vi "Pilot-Screen.vi"() -> ()   [LabVIEW 2018]
uses:
  <vilib>/userdefined/High Color/IMAQdx.ctl
  <vilib>/vision/Shape Detection.llb/ShapeDetectionMatchOptions.ctl
  <vilib>/vision/Pattern Matching.llb/IMAQ Match Range Setting.ctl
  <vilib>/express/express arith-compare/Formula/XNode/ExpressFormulaBlockNode.xnode
  <vilib>/vision/driver/NI_Vision_Acquisition_Software.lvlib
  <vilib>/MakerHub/LINX/LMH-LINX.lvlib
  <vilib>/vision/NI_Vision_Development_Module.lvlib
panel:
  in  "Tab Control":enum32{"Cannon calculations", "Shape Detection"}(tab)
  out "lift capability of ROV":dbl format="%#.1f"
  out "String 8":string
  in  "Cannon Volume":dbl format="%#.1f"
  out "Scaled Distance":dbl format="%#.1f"
  in  "Real Distance":dbl format="%#_6f"
  in  "Set Refrence":bool
  in  "Stop 2":bool
  out "Cannon Weight":dbl format="%#.1f"
  out "String 6":string
  out "String 7":string
  in  "Composition":u16(ring) items=["Select"=0, "AF"=8030, "Else"=7870]
  out "ROV Can Lift?":bool
  out "Snapshot":T1(plugin-control)
  out "String":string
  out "String 2":string
  out "String 4":string
  out "String 5":string
  in  "R1 2":dbl format="%#.1f"
  in  "R2 2":dbl format="%#.1f"
  in  "R3 2":dbl format="%#.1f"
  in  "L 2":bool
  in  "R1":bool
  in  "R2":bool
  in  "R3":bool
  in  "L":dbl format="%#.1f"
  out "Snapshot 2":T1(plugin-control)
  out "Done":bool
  out "Lines":i32
  out "Triangles":i32
  out "Squares":i32
  out "Circles":i32
  out "Objects":i32
  in  "Start Detecting":bool
  out "measurment Video":T1(plugin-control)
  in  "Scaled Pixels":dbl
  in  "Real Pixels":dbl
  in  "measurment camera":T2
  in  "Stop":bool
  in  "Gribber":T2="cam7"
  out "Loop Rate (Hz)":u32
  out "Grebber Camera":T1(plugin-control)
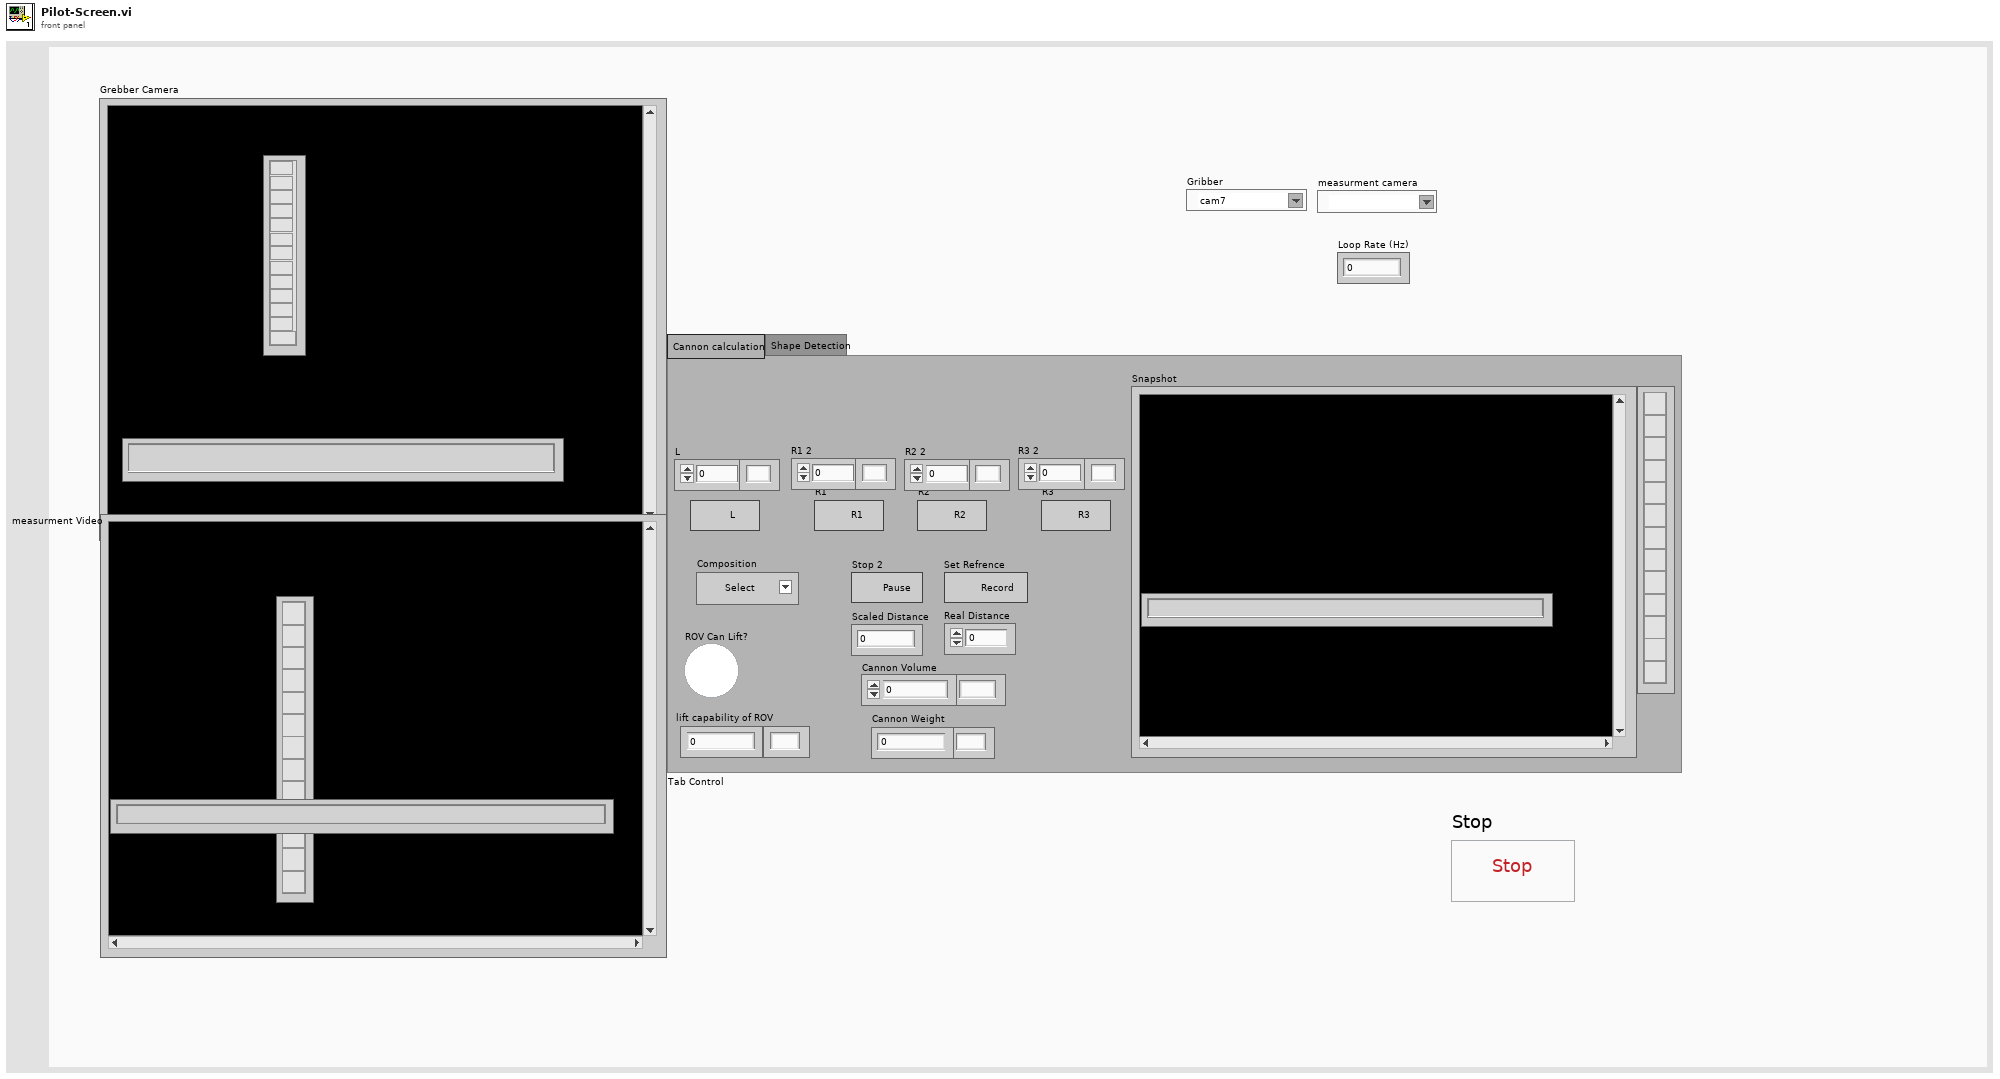
[diagram p1: front panel]
types:
  T1 = typedef "IMAQ Image.ctl" = refnum<image>
  T2 = typedef "IMAQdx.ctl" = refnum<k21>
  T3 = typedef "Image Type" = u32
  T4 = typedef "ShapeDetectionMatchOptions.ctl" = cluster{"Rotation":bool, "Scale":bool, "Occlusion":bool, "Range Settings":T5[]}
  T5 = typedef "IMAQ Match Range Setting.ctl" = cluster{"Match Constraints":u32, "Min":dbl, "Max":dbl}
  T6 = cluster{"Objects":u16, "Threshold":i32, "Reject Border":bool, "Fill Holes":bool, "Min Object Size":bool, "Min Size":i32, "Max Object Size":bool, "Max Size":i32, "Show Search Area":bool, "Show Center":bool, "Show Bounding Box":bool}
  T7 = cluster{"Global Rectangle":i32[], "Contours":cluster{"Contour Type":u32, "ROI Type":u32, "Points":i32[]}[]}
  T8 = typedef "IMAQ Line" = cluster{"Start X":i32, "Start Y":i32, "End X":i32, "End Y":i32}
  T9 = typedef "IMAQ Rectangle" = cluster{"Left":i32, "Top":i32, "Right":i32, "Bottom":i32, "Rotation":dbl}
  T10 = cluster{"Object Center":cluster{"X":sgl, "Y":sgl}, "Bounding Box":cluster{"X Left":i32, "Y Top":i32, "X Right":i32, "Y Bottom":i32}, "Area":sgl, "Orientation":sgl, "Aspect Ratio":sgl, "Nb Holes":i32}[]
  T11 = cluster{"Object Center":cluster{"X":sgl, "Y":sgl}, "Bounding Box":cluster{"X Left":i32, "Y Top":i32, "X Right":i32, "Y Bottom":i32}, "Area":sgl, "Orientation":sgl, "Aspect Ratio":sgl, "Nb Holes":i32}
  T12 = typedef "ROI Descriptor" = cluster{"Global Rectangle":i32[], "Contours":cluster{"ID":enum32{"External", "Internal"}, "Type":u32, "Coordinates":i32[]}[]}
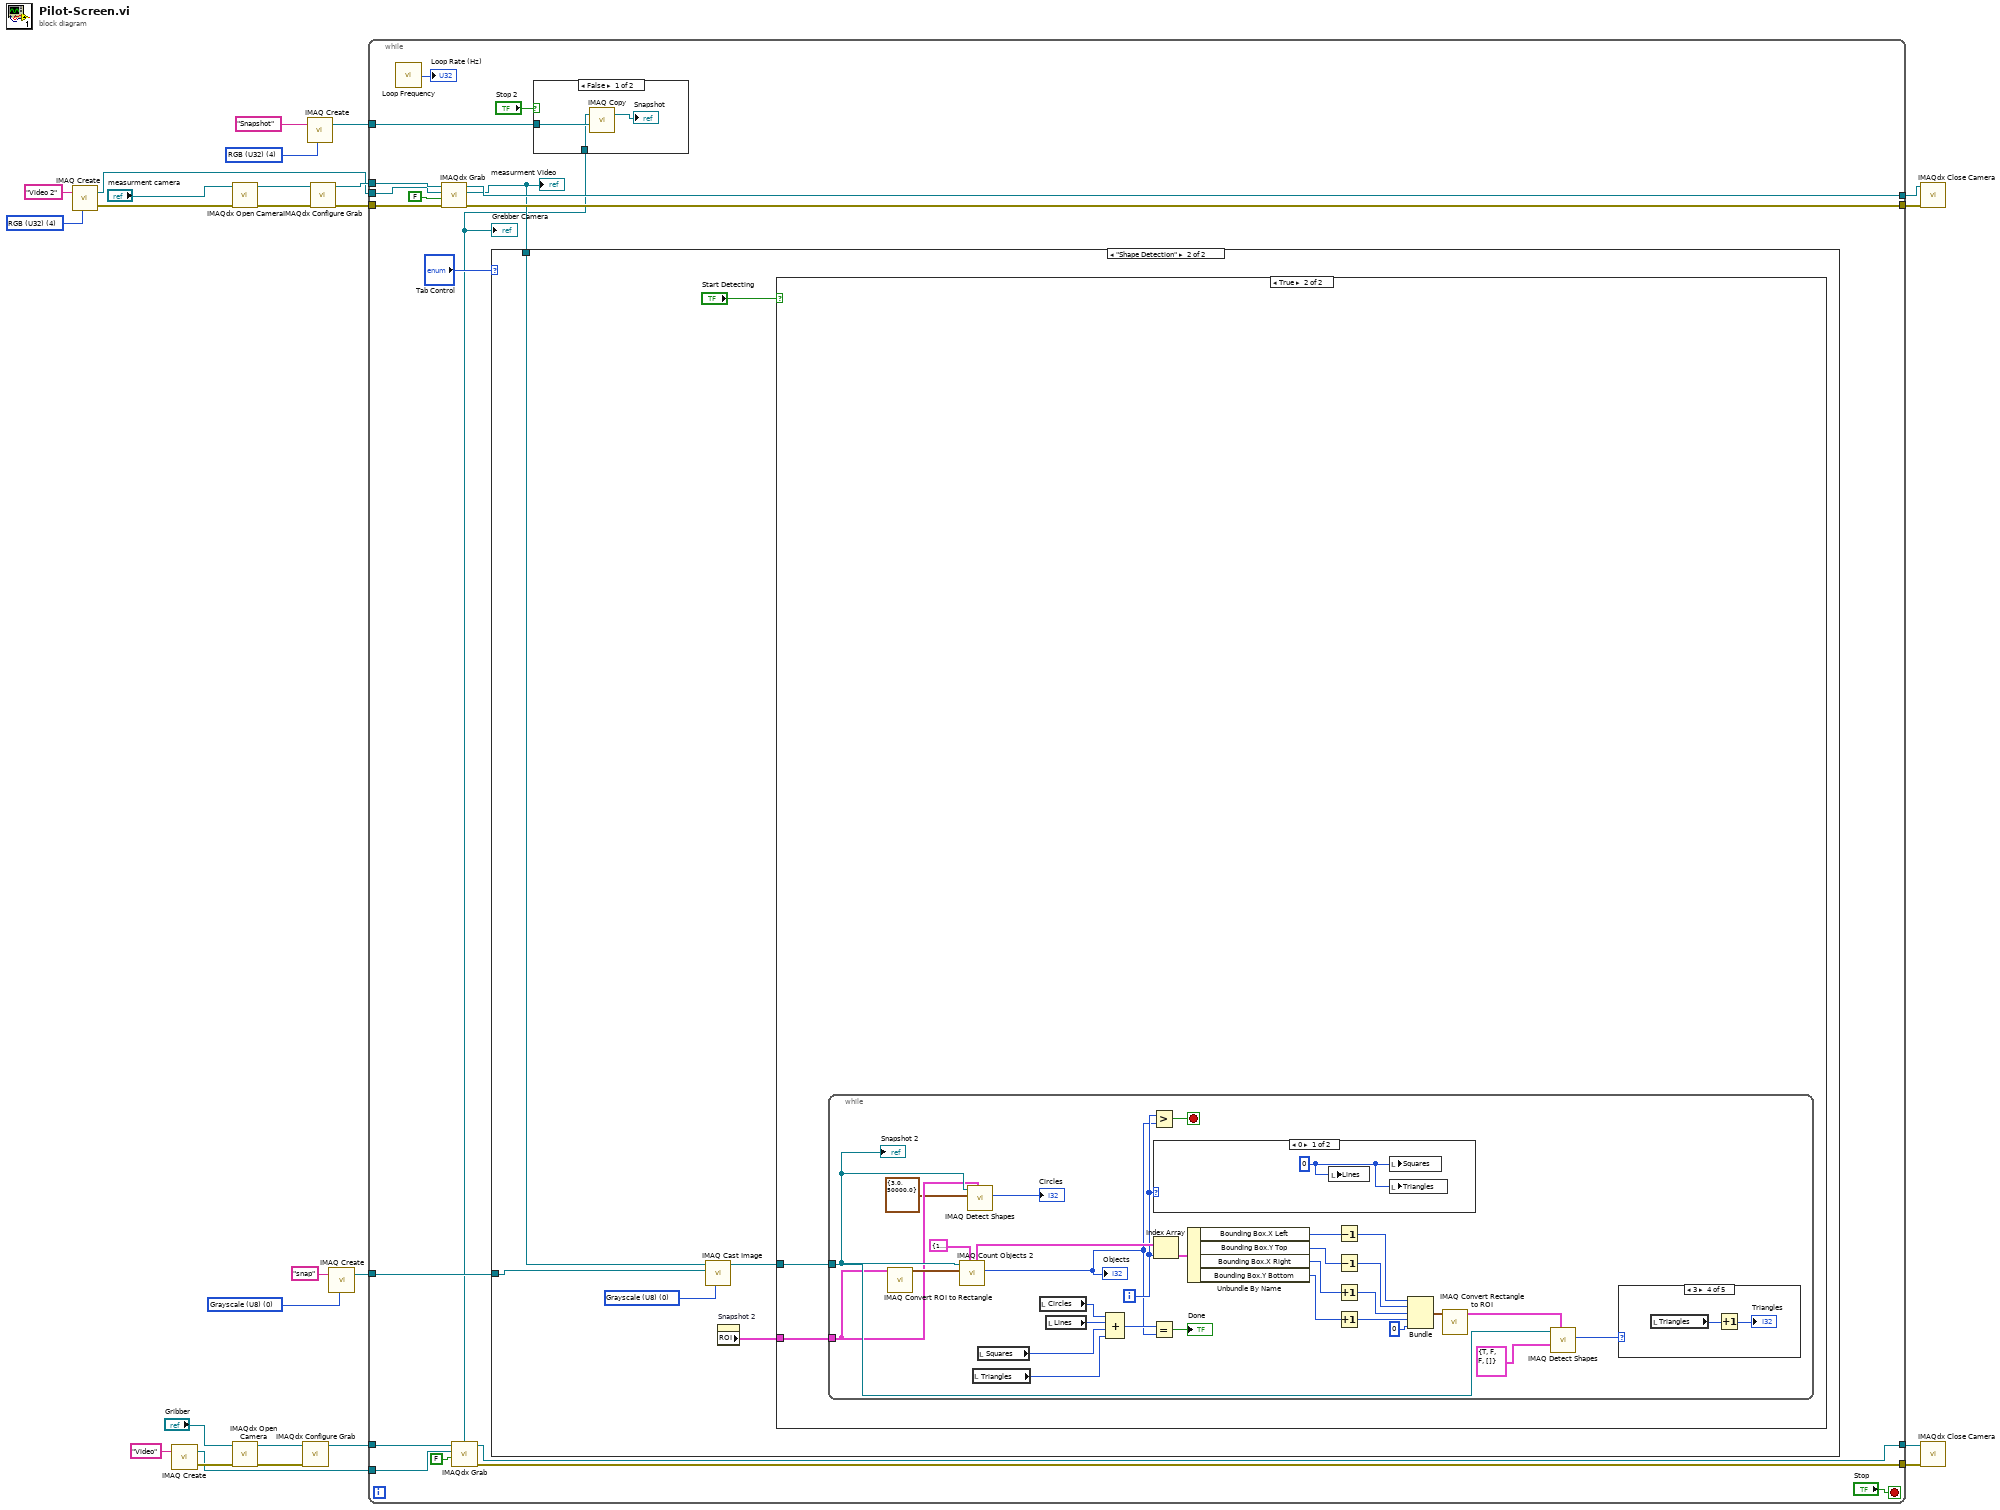
[diagram p0: block diagram]
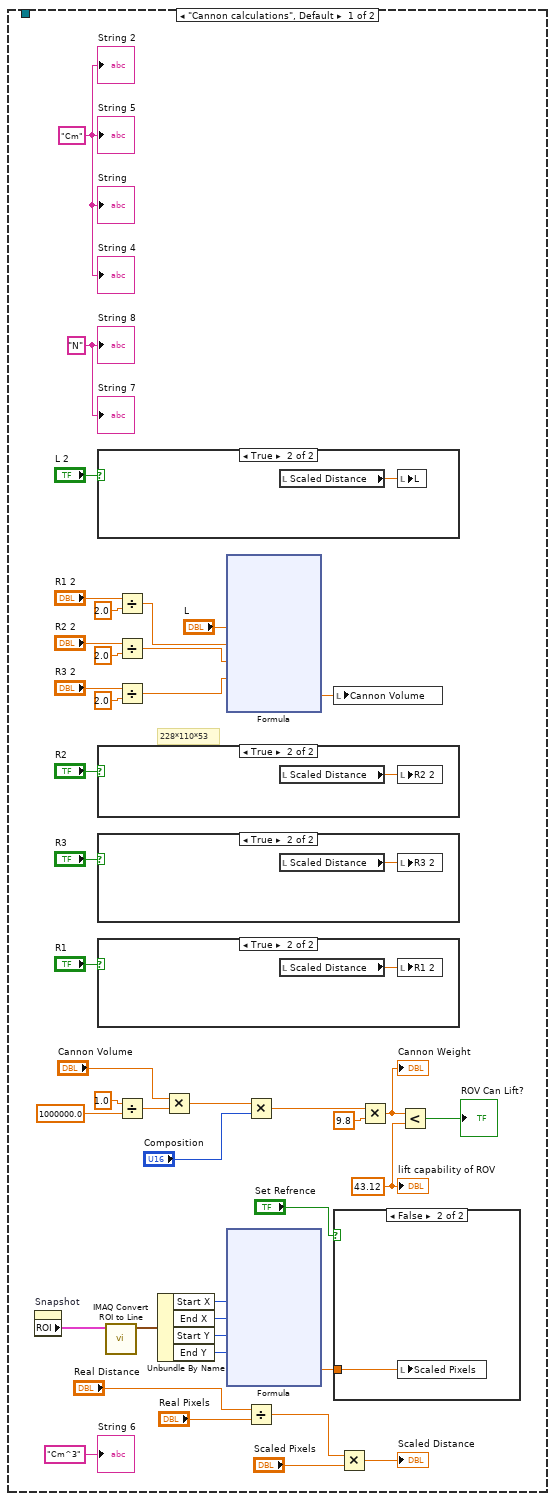
[diagram p2: hidden frame]
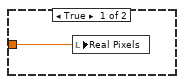
[diagram p7: hidden frame]
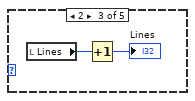
[diagram p11: hidden frame]
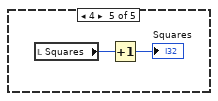
[diagram p12: hidden frame]
diagram:
  w3 = T3 0 items=["Grayscale (U8)", "Grayscale (I16)", "Grayscale (SGL)", "Complex (CSG)", "RGB (U32)", "HSL (U32)", "RGB (U64)", "Grayscale (U16)"] ("Image Type")
  w15 = T3 4 items=["Grayscale (U8)", "Grayscale (I16)", "Grayscale (SGL)", "Complex (CSG)", "RGB (U32)", "HSL (U32)", "RGB (U64)", "Grayscale (U16)"] ("Image Type")
  w13 = T3 4 items=["Grayscale (U8)", "Grayscale (I16)", "Grayscale (SGL)", "Complex (CSG)", "RGB (U32)", "HSL (U32)", "RGB (U64)", "Grayscale (U16)"] ("Image Type")
  n1 = call "IMAQ Create"("Image Name"="Video 2", "Image Type"=w13) -> ("New Image"=w8:T1, "error out"=w17:errorcluster)  [unwired: 2 in, 1 out]
  n2 = call "IMAQ Create"("Image Name"="Video") -> ("New Image"=w22:T1, "error out"=w26:errorcluster)  [unwired: 3 in, 1 out]
  n3 = call <vilib>:"IMAQdx Open Camera.vi"("error in"=w17, "Session In"="measurment camera") -> ("error out"=w12:errorcluster, "Session Out"=w11:T2)  [unwired: 8 in]
  n4 = call <vilib>:"IMAQdx Open Camera.vi"("error in"=w26, "Session In"="Gribber") -> ("error out"=w25:errorcluster, "Session Out"=w24:T2)  [unwired: 8 in]
  n5 = call <vilib>:"IMAQdx Configure Grab.vi"("error in"=w25, "Session In"=w24) -> ("Session Out"=w21:T2)  [unwired: 8 in, 1 out]
  n6 = call "IMAQ Create"("Image Name"="Snapshot", "Image Type"=w15) -> ("New Image"=w7:T1)  [unwired: 3 in, 1 out]
  n7 = call <vilib>:"IMAQdx Configure Grab.vi"("error in"=w12, "Session In"=w11) -> ("error out"=w9:errorcluster, "Session Out"=w10:T2)  [unwired: 8 in]
  n8 = call "IMAQ Create"("Image Name"="snap", "Image Type"=w3) -> ("New Image"=w1:T1)  [unwired: 2 in, 2 out]
  n9 = while {
    tunnel: w22 -> [w45]
    tunnel: w21 -> [w44]
    tunnel: [w43] -> w20
    tunnel: w10 -> [w39]
    tunnel: w9 -> [w38]
    tunnel: w8 -> [w37]
    tunnel: w7 -> [w36]
    tunnel: [w34] -> w6
    tunnel: [w33] -> w5
    tunnel: [w32] -> w4
    tunnel: w1 -> [w29]
    stop <- "Stop" stop-if-true
    n10 = call <vilib>:"Loop Frequency.vi"() -> ("Loop Rate (Hz)"=→"Loop Rate (Hz)":u32)
    n11 = call <vilib>:"IMAQdx Grab.vi"("error in"=w38, "Wait for Next Buffer? (Yes)"=FALSE, "Image In"=w37, "Session In"=w39) -> ("error out"=w33:errorcluster, "Image Out"=w28:T1, "Session Out"=w34:T2)  [unwired: 5 out]
    "measurment Video" <- w28
    n12 = call <vilib>:"IMAQdx Grab.vi"("Wait for Next Buffer? (Yes)"=FALSE, "Image In"=w45, "Session In"=w44) -> ("error out"=w32:errorcluster, "Image Out"=w27:T1, "Session Out"=w43:T2)  [unwired: 1 in, 5 out]
    "Grebber Camera" <- w27
    n13 = case shown="\"Shape Detection\"" "Tab Control" {
      tunnel: w29 -> [_ w125]
      tunnel: w28 -> [_ w122]
      frame "Cannon calculations", Default {
        w46 = "N" ("String 6")
        w60 = 43.12 ("y")
        w56 = "Cm"
        # "228*110*53"
        n14 = property on="Snapshot" class="ImageControl"() -> ("ROI"=w68:T7)  [unwired: 2 in, 2 out]
        n15 = case shown="True" "L 2" {
          frame False {
          }
          frame True {
            n16 = local read "Scaled Distance"() -> (w88:dbl)
            n17 = local write "L"(w88) -> ()
          }
        }
        n18 = case shown="True" "R2" {
          frame False {
          }
          frame True {
            n19 = local read "Scaled Distance"() -> (w90:dbl)
            n20 = local write "R2 2"(w90) -> ()
          }
        }
        n21 = case shown="True" "R3" {
          frame False {
          }
          frame True {
            n22 = local read "Scaled Distance"() -> (w91:dbl)
            n23 = local write "R3 2"(w91) -> ()
          }
        }
        n24 = case shown="True" "R1" {
          frame False {
          }
          frame True {
            n25 = local read "Scaled Distance"() -> (w89:dbl)
            n26 = local write "R1 2"(w89) -> ()
          }
        }
        n27 = call "IMAQ Convert ROI to Line"("ROI Descriptor"=w68) -> ("Line"=w67:T8)  [unwired: 8 in, 1 out]
        n28 = Divide(x="R1 2", y=2.0) -> (x/y=w80:dbl)
        n29 = Divide(x="R2 2", y=2.0) -> (x/y=w82:dbl)
        n30 = Divide(x="R3 2", y=2.0) -> (x/y=w83:dbl)
        n31 = Divide(x=1.0, y=1000000.0) -> (x/y=w76:dbl)
        n32 = Unbundle By Name(w67) -> ("Start X"=w63:i32, "End X"=w64:i32, "Start Y"=w65:i32, "End Y"=w66:i32)
        n33 = Multiply(x="Cannon Volume", y=w76) -> (x*y=w75:dbl)
        n34 = xnode "Formula"("L"="L", "R1"=w80, "R2"=w82, "R3"=w83) -> ("Result"=w77:dbl)  [unwired: 1 in, 1 out]
        n35 = xnode ("Formula")("Start X"=w63, "End X"=w64, "Start Y"=w65, "End Y"=w66) -> ("Result"=w69:dbl)  [unwired: 1 in, 1 out]
        n36 = Multiply(x=w75, y="Composition") -> (x*y=w74:dbl)
        n37 = Divide(x="Real Distance", y="Real Pixels") -> (x/y=w50:dbl)
        n38 = local write "Cannon Volume"(w77) -> ()
        n39 = case shown="False" "Set Refrence" {
          tunnel: w69 -> [w106 w107]
          frame True {
            n40 = local write "Real Pixels"(w106) -> ()
          }
          frame False {
            n41 = local write "Scaled Pixels"(w107) -> ()
          }
        }
        n42 = Multiply(x=w50, y="Scaled Pixels") -> (x*y=→"Scaled Distance":dbl)
        n43 = Multiply(x=w74, y=9.8) -> (x*y=w86:dbl)
        "Cannon Weight" <- w86
        n44 = Less?(x=w86, y=w60) -> (x < y?=→"ROV Can Lift?":bool)
        "String 6" <- "Cm^3" ("String 6")
        "String" <- w56
        "String 2" <- w56
        "String 4" <- w56
        "String 5" <- w56
        "lift capability of ROV" <- w60
        "String 8" <- w46
        "String 7" <- w46
      }
      frame "Shape Detection" {
        w127 = T3 0 items=["Grayscale (U8)", "Grayscale (I16)", "Grayscale (SGL)", "Complex (CSG)", "RGB (U32)", "HSL (U32)", "RGB (U64)", "Grayscale (U16)"] ("Image Type")
        n45 = call "IMAQ Cast Image"("Image Type"=w127, "Image Dst"=w125, "Image Src"=w122) -> ("Image Dst Out"=w126:T1)  [unwired: 7 in, 1 out]
        n46 = property on="Snapshot 2" class="ImageControl"() -> ("ROI"=w123:T7)  [unwired: 2 in, 2 out]
        n47 = case shown="True" "Start Detecting" {
          tunnel: w126 -> [_ w129]
          tunnel: w123 -> [_ w128]
          frame False {
          }
          frame True {
            n48 = while {
              tunnel: w129 -> [w133]
              tunnel: w128 -> [w131]
              i -> [w142]
              stop <- w141 stop-if-true
              n49 = call "IMAQ Convert ROI to Rectangle"("ROI Descriptor"=w131) -> ("Rectangle"=w132:T9)  [unwired: 8 in, 1 out]
              n50 = call "IMAQ Count Objects 2"("Settings"=T6 {"Objects"=1, "Threshold"=100, "Reject Border"=TRUE, "Fill Holes"=FALSE, "Min Object Size"=TRUE, "Min Size"=300, "Max Object Size"=FALSE, "Max Size"=100, "Show Search Area"=FALSE, "Show Center"=TRUE, "Show Bounding Box"=TRUE}, "Search Rect (entire image)"=w132, "Image"=w133) -> ("Number of Objects"=w135:i32, "Objects"=w158:T10)  [unwired: 4 in, 3 out]
              "Objects" <- w135
              n51 = call-poly "IMAQ Detect Shapes"("ROI Descriptor"=w131, "Circle Descriptor"=cluster{"Min Radius":dbl, "Max Radius":dbl} {"Min Radius"=3.0, "Max Radius"=50000.0}, "Image"=w133) -> ("Number of Matches Returned"=→"Circles":i32)  [unwired: 6 in, 2 out]
              n52 = local read "Triangles"() -> (w137:i32)
              n53 = local read "Squares"() -> (w138:i32)
              n54 = local read "Circles"() -> (w140:i32)
              n55 = local read "Lines"() -> (w139:i32)
              n56 = Compound Arithmetic op=ADD(w140, w139, w138, w137) -> (w136:i32)
              n57 = Greater?(x=w142, y=w135) -> (0:w141:bool)
              n58 = Equal?(x=w136, y=w135) -> (x = y?=→"Done":bool)
              n59 = case shown="0" w142 {
                frame 0 {
                  w166 = 0
                  n60 = local write "Lines"(w166) -> ()
                  n61 = local write "Squares"(w166) -> ()
                  n62 = local write "Triangles"(w166) -> ()
                }
                frame 1, Default {
                }
              }
              n63 = Index Array(array=w158, index=w142) -> (element=w156:T11)
              n64 = Unbundle By Name(w156) -> ("Bounding Box.X Left"=w153:i32, "Bounding Box.Y Top"=w152:i32, "Bounding Box.X Right"=w151:i32, "Bounding Box.Y Bottom"=w150:i32)
              n65 = Decrement(x=w153) -> (x-1=w149:i32)
              n66 = Decrement(x=w152) -> (x-1=w148:i32)
              n67 = Increment(x=w151) -> (x+1=w147:i32)
              n68 = Increment(x=w150) -> (x+1=w146:i32)
              n69 = Bundle(w149, w148, w147, w146, "index"=0) -> (w145:cluster{i32, i32, i32, i32, "index":i32})  [unwired: 1 in]
              n70 = call "IMAQ Convert Rectangle to ROI"("Rectangle"=w145) -> ("ROI Descriptor"=w154:T12)  [unwired: 8 in, 1 out]
              n71 = call-poly "IMAQ Detect Shapes"("ROI Descriptor"=w154, "Match Options"=T4 {"Rotation"=TRUE, "Scale"=FALSE, "Occlusion"=FALSE, "Range Settings"=[]}, "Image"=w133) -> ("Number of Matches Returned"=w143:i32)  [unwired: 6 in, 2 out]
              n72 = case shown="3" w143 {
                frame 0, Default {
                }
                frame 1 {
                }
                frame 2 {
                  n73 = local read "Lines"() -> (w161:i32)
                  n74 = Increment(x=w161) -> (x+1=→"Lines":i32)
                }
                frame 3 {
                  n75 = local read "Triangles"() -> (w163:i32)
                  n76 = Increment(x=w163) -> (x+1=→"Triangles":i32)
                }
                frame 4 {
                  n77 = local read "Squares"() -> (w165:i32)
                  n78 = Increment(x=w165) -> (x+1=→"Squares":i32)
                }
              }
              "Snapshot 2" <- w133
            }
          }
        }
      }
    }
    n79 = case shown="False" "Stop 2" {
      tunnel: w36 -> [w168 _]
      tunnel: w27 -> [w167 _]
      frame False {
        n80 = call "IMAQ Copy"("Image Dst"=w168, "Image Src"=w167) -> ("Image Dst Out"=→"Snapshot":T1)  [unwired: 4 in, 1 out]
      }
      frame True {
      }
    }
  }
  n81 = call <vilib>:"IMAQdx Close Camera.vi"("error in"=w5, "Session In"=w6) -> ()  [unwired: 10 out]
  n82 = call <vilib>:"IMAQdx Close Camera.vi"("error in"=w4, "Session In"=w20) -> ()  [unwired: 10 out]
